vi "Test Suite Result Pass Count.vi"(8 "error in (no error)":errorcluster, 11 "Test Suite Result Test In":refnum<class "Test Suite Result Test.lvclass">) -> (0 "error out":errorcluster, 3 "Test Suite Result Test Out":refnum<class "Test Suite Result Test.lvclass">)   [LabVIEW 2020, in "LUnit Tests.lvlib" / "Test Suite Result Test.lvclass"]
uses:
  Test Suite Result Test.lvclass
  source/Examples/Basic Example/Passing Test Case/Passing Test Case.lvclass
  40130bf0-0af1-4eb8-8735-7f61a2509a7e.vi
  source/Framework/Result Types/Assertion Result/Public/TypeDefs/Status.ctl
  source/Framework/Result Types/Assertion Result/Assertion Result.lvlib
  source/Framework/Result Types/Case Result/Test Case Result.lvlib
  C:/Git/astemes-lunit/source/Framework/Test Case/LUnit Test Case.lvclass
  C:/Git/astemes-lunit/source/Examples/Basic Example/Passing Test Case/Passing Test Case.lvclass
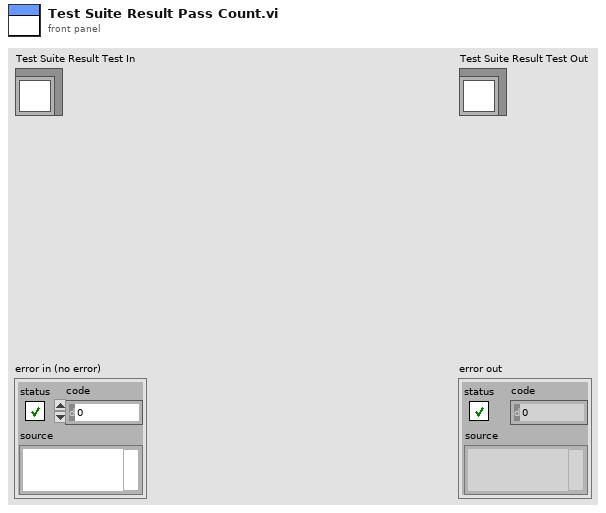
[diagram p1: front panel]
types:
  T1 = typedef "Assertion Result.lvlib/Status.ctl" = enum16{"Pass", "Fail", "Error", "Skipped", "Setup Error", "Broken", "Teardown Error"}
  T2 = typedef "Test Suite Result.lvlib/Test Suite Result.ctl" = cluster{"Test Suite ID":string, "Name":string, "Hostname":string, "Status":T1, "Execution time":dbl, "Start Time":timestamp, "Case Results":T3[]}
  T3 = typedef "Test Case Result.lvlib/Test Case Result.ctl" = map{string, T4}
  T4 = typedef "Method Result.lvlib/Method Result.ctl" = cluster{"Test Case":string, "Test Method Name":string, "Status":T1, "Assertion Results":T5[], "Execution time":dbl, "Result String":string}
  T5 = typedef "Assertion Result.lvlib/Assertion Result.ctl" = cluster{"Status":T1, "Message":string, "Description":string, "Assertion Type":T6}
  T6 = typedef "Assertion Result.lvlib/Assertion Type.ctl" = enum16{"None", "Pass", "Fail", "Skip", "Pass if Equal", "Fail if Equal", "Pass if Error", "Fail if Error", "Pass if", "Fail if"}
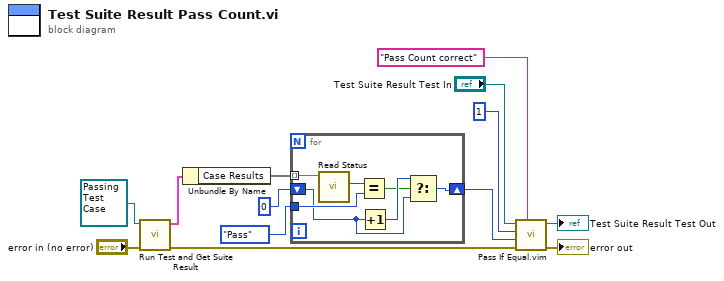
[diagram p0: block diagram]
diagram:
  n1 = call "Run Test and Get Suite Result.vi"("error in (no error)"="error in (no error)", "Test Test Case in"=refnum<class "Passing Test Case.lvclass"> refnum ("Passing Test Case.lvclass")) -> ("error out"=w7:errorcluster, "Test Suite Result out"=w3:T2)  [unwired: 8 in]
  n2 = Unbundle By Name(w3) -> ("Case Results"=w2:T3[])
  n3 = for {
    tunnel: w2 -> [w20] mode=indexing
    tunnel: Status."Pass" ("Status") -> [w18]
    shift-right: [w15] -> w12
    shift-left: 0 -> [w16]
    n4 = call "Read Status.vi"("Test Case Result In"=w20) -> ("Status"=w19:T1)  [unwired: 8 in, 2 out]
    n5 = Equal?(x=w19, y=w18) -> (x = y?=w14:bool)
    n6 = Increment(x=w16) -> (x+1=w17:i32)
    n7 = Select(t=w17, s=w14, f=w16) -> (s? t:f=w15:i32)
  }
  n8 = call "Pass If Equal.vim"("Description"="Pass Count correct", "error in (no error)"=w7, "Actual"=w12, "Expected"=1 ("x"), "LUnit Test Case In"="Test Suite Result Test In") -> ("error out"=→"error out":errorcluster, "LUnit Test Case Out"=→"Test Suite Result Test Out":refnum<class "Test Suite Result Test.lvclass">)  [unwired: 5 in]
